vi "OEE_PART_2_P.vi"(0 "Refnum in":T1, 1 "Shift":string, 3 "String":string, 5 "Select Station":string, 9 "Form Date":timestamp, 11 "To Date":timestamp, 12 "AVAILABLILITY TIME":dbl, 14 "CAPACITY":dbl) -> (4 "Refnum out":T1, 6 "Array":string[][](array[string]), 8 "QUALITY":dbl, 10 "Production count":i32, 13 "OEE":dbl format="%#_3g", 15 "PERFORMANCE":dbl)   [LabVIEW 2017]
uses:
  <vilib>/addons/database/Connection.llb/Conn ObjectReference.ctl
  <vilib>/addons/database/NI_Database_API.lvlib
panel:
  out "ALL IN ONE":string[][](array[string])
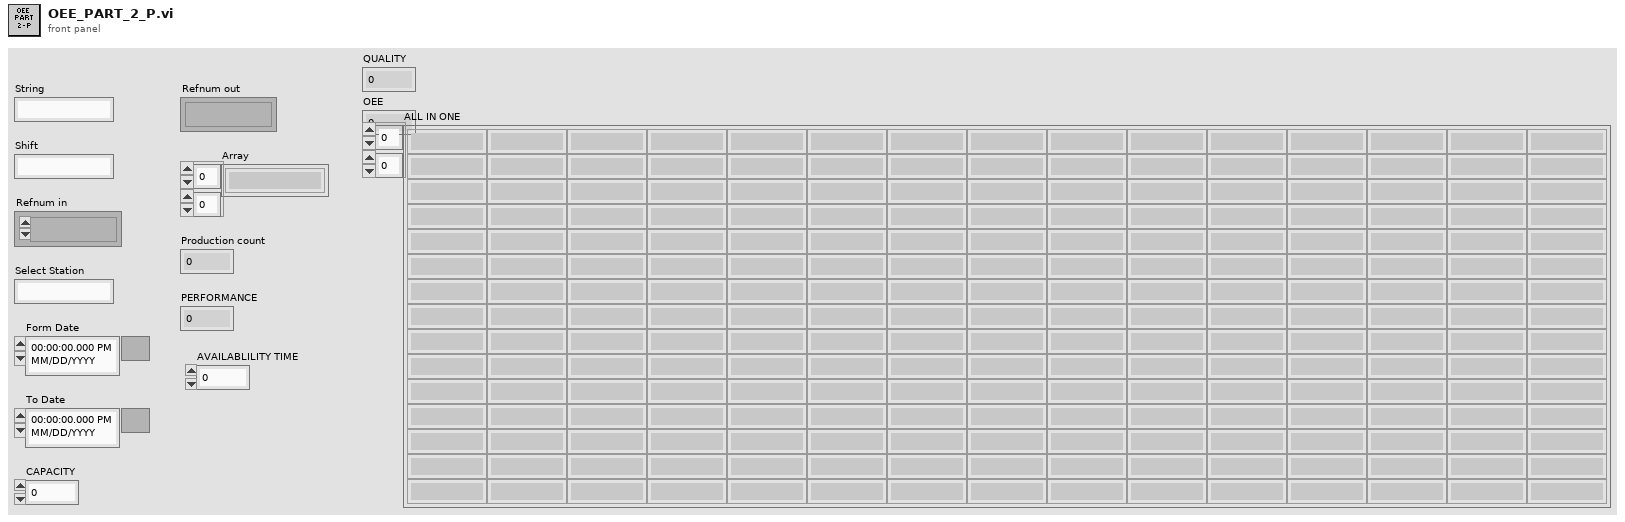
[diagram p1: front panel]
types:
  T1 = typedef "NI_Database_API.lvlib/Conn ObjectReference.ctl" = refnum<k1>
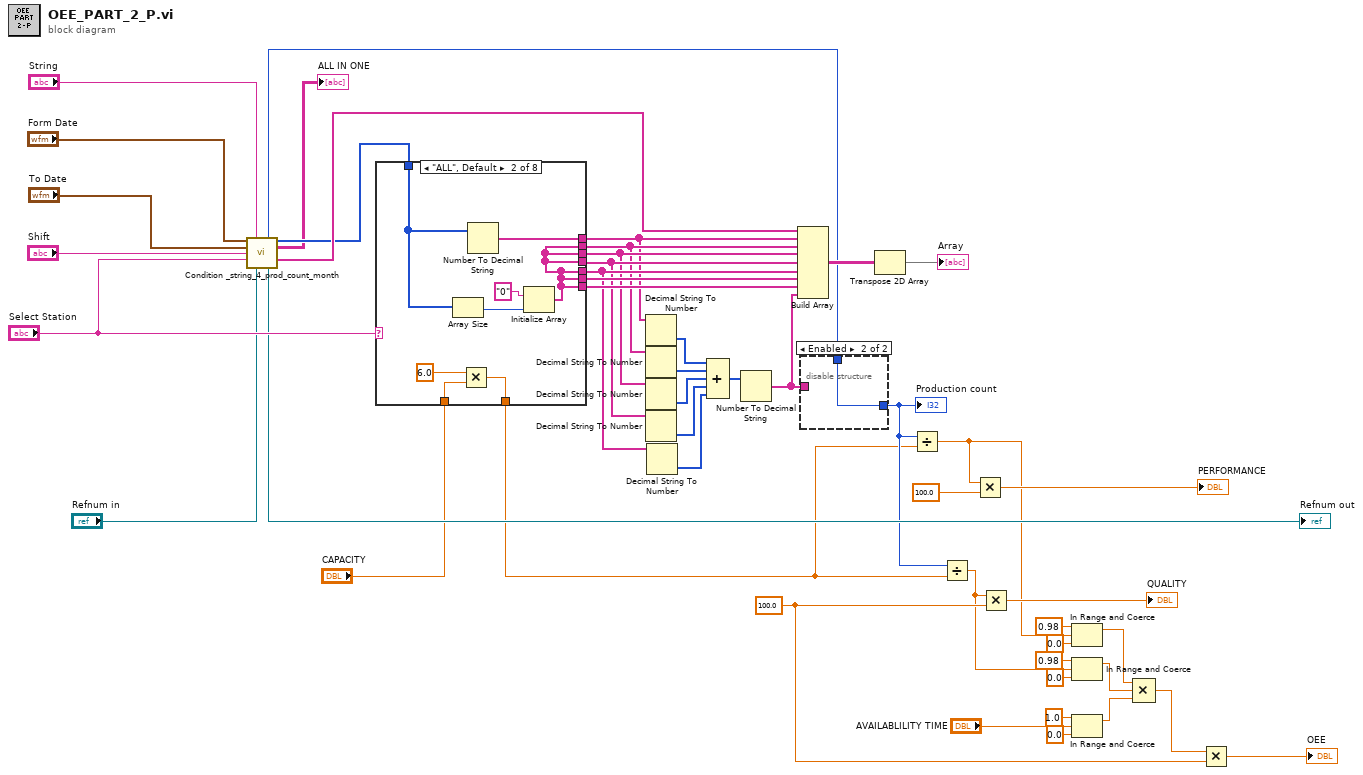
[diagram p0: block diagram]
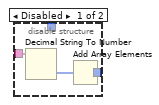
[diagram p2: hidden frame]
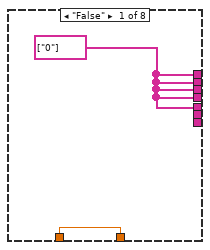
[diagram p3: hidden frame]
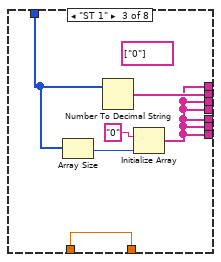
[diagram p4: hidden frame]
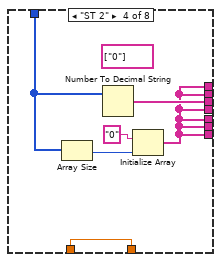
[diagram p5: hidden frame]
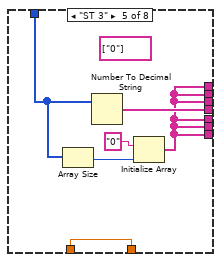
[diagram p6: hidden frame]
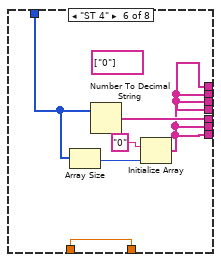
[diagram p7: hidden frame]
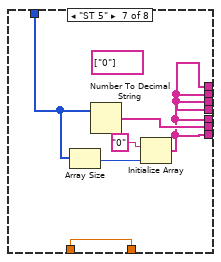
[diagram p8: hidden frame]
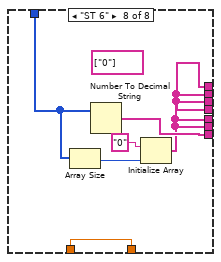
[diagram p9: hidden frame]
diagram:
  w18 = 100.0 ("y")
  n1 = call "Condition _string_4_prod_count_month.vi"("From Date"="Form Date", "Select Stakeholder"="String", "To Date"="To Date", "Shift"="Shift", "Select Station"="Select Station", "Refnum out 2"="Refnum in") -> ("Count"=w15:i32, "sum"=w39:i32[], "ALL IN ONE"=→"ALL IN ONE":string[][], "Elements Found out"=w40:string[], "Refnum out"=→"Refnum out":T1)  [unwired: 2 in, 3 out]
  n2 = case shown="\"ALL\", Default" "Select Station" {
    tunnel: w39 -> [_ w57 w61 w67 w73 w79 w86 w92]
    tunnel: [w50 w58 w60 w66 w72 w78 w84 w90] -> w31
    tunnel: [w50 w54 w64 w66 w72 w78 w84 w90] -> w32
    tunnel: [w50 w54 w60 w70 w72 w78 w84 w90] -> w33
    tunnel: [w50 w54 w60 w66 w76 w78 w84 w90] -> w34
    tunnel: [w50 w54 w60 w66 w72 w82 w84 w90] -> w35
    tunnel: [_ w54 w60 w66 w72 w78 w85 w90] -> w37
    tunnel: [_ w54 w60 w66 w72 w78 w84 w91] -> w38
    tunnel: [w49 w51 w59 w65 w71 w77 w83 w89] -> w13
    tunnel: "CAPACITY" -> [w49 w52 w59 w65 w71 w77 w83 w89]
    frame "False" {
      w50 = string[] ["0"]
    }
    frame "ALL", Default {
      n3 = Array Size(array=w57) -> (size(s)=w56:i32)
      n4 = Multiply(x=6.0, y=w52) -> (x*y=w51:dbl)
      n5 = Number To Decimal String(number=w57) -> (decimal integer string=w58:string[])  [unwired: 1 in]
      n6 = Initialize Array("0", w56) -> (w54:string[])
    }
    frame "ST 1" {
      (unwired) string[] ["0"]
      n7 = Array Size(array=w61) -> (size(s)=w63:i32)
      n8 = Number To Decimal String(number=w61) -> (decimal integer string=w64:string[])  [unwired: 1 in]
      n9 = Initialize Array("0", w63) -> (w60:string[])
    }
    frame "ST 2" {
      (unwired) string[] ["0"]
      n10 = Array Size(array=w67) -> (size(s)=w69:i32)
      n11 = Number To Decimal String(number=w67) -> (decimal integer string=w70:string[])  [unwired: 1 in]
      n12 = Initialize Array("0", w69) -> (w66:string[])
    }
    frame "ST 3" {
      (unwired) string[] ["0"]
      n13 = Array Size(array=w73) -> (size(s)=w75:i32)
      n14 = Number To Decimal String(number=w73) -> (decimal integer string=w76:string[])  [unwired: 1 in]
      n15 = Initialize Array("0", w75) -> (w72:string[])
    }
    frame "ST 4" {
      (unwired) string[] ["0"]
      n16 = Array Size(array=w79) -> (size(s)=w81:i32)
      n17 = Number To Decimal String(number=w79) -> (decimal integer string=w82:string[])  [unwired: 1 in]
      n18 = Initialize Array("0", w81) -> (w78:string[])
    }
    frame "ST 5" {
      (unwired) string[] ["0"]
      n19 = Array Size(array=w86) -> (size(s)=w88:i32)
      n20 = Number To Decimal String(number=w86) -> (decimal integer string=w85:string[])  [unwired: 1 in]
      n21 = Initialize Array("0", w88) -> (w84:string[])
    }
    frame "ST 6" {
      (unwired) string[] ["0"]
      n22 = Array Size(array=w92) -> (size(s)=w94:i32)
      n23 = Number To Decimal String(number=w92) -> (decimal integer string=w91:string[])  [unwired: 1 in]
      n24 = Initialize Array("0", w94) -> (w90:string[])
    }
  }
  n25 = Decimal String To Number(string=w31) -> (number=w30:i32[])  [unwired: 2 in, 1 out]
  n26 = Decimal String To Number(string=w32) -> (number=w29:i32[])  [unwired: 2 in, 1 out]
  n27 = Decimal String To Number(string=w33) -> (number=w28:i32[])  [unwired: 2 in, 1 out]
  n28 = Decimal String To Number(string=w34) -> (number=w27:i32[])  [unwired: 2 in, 1 out]
  n29 = Decimal String To Number(string=w35) -> (number=w36:i32[])  [unwired: 2 in, 1 out]
  n30 = Compound Arithmetic op=ADD(w30, w29, w28, w27, w36) -> (w26:i32[])
  n31 = Number To Decimal String(number=w26) -> (decimal integer string=w42:string[])  [unwired: 1 in]
  n32 = Build Array(w40, w31, w32, w33, w34, w35, w37, w38, w42) -> (w25:string[][])
  n33 = disable-structure shown="Enabled" {
    disable-tunnel: w42 -> [w96 _]
    disable-tunnel: [w95 w98] -> w22
    disable-tunnel: w15 -> [_ w98]
    frame Disabled {
      n34 = Decimal String To Number(string=w96) -> (number=w97:i32[])  [unwired: 2 in, 1 out]
      n35 = Add Array Elements(numeric array=w97) -> (sum=w95:i32)
    }
    frame Enabled {
    }
  }
  "Production count" <- w22
  n36 = Transpose 2D Array(2D array=w25) -> (transposed array=→"Array":string[][])
  n37 = Divide(x=w22, y=w13) -> (x/y=w10:dbl)
  n38 = Divide(x=w22, y=w13) -> (x/y=w6:dbl)
  n39 = Multiply(x=w10, y=100.0) -> (x*y=→"PERFORMANCE":dbl)
  n40 = Multiply(x=w6, y=w18) -> (x*y=→"QUALITY":dbl)
  n41 = In Range and Coerce(upper limit=0.98, x=w10, lower limit=0.0) -> (coerced(x)=w9:dbl)  [unwired: 1 out]
  n42 = In Range and Coerce(upper limit=0.98, x=w6, lower limit=0.0) -> (coerced(x)=w5:dbl)  [unwired: 1 out]
  n43 = In Range and Coerce(upper limit=1.0, x="AVAILABLILITY TIME", lower limit=0.0) -> (coerced(x)=w1:dbl)  [unwired: 1 out]
  n44 = Compound Arithmetic op=MULTIPLY(w9, w5, w1) -> (w19:dbl)
  n45 = Multiply(x=w19, y=w18) -> (x*y=→"OEE":dbl)
